vi "combine clusters (SubVI).vi"(10 "Output Configuration":T1[](array[typedef]) {"boolean high" format="%#_17g"; "boolean low" format="%#_17g"; "scan step" format="%#_17g"; "scan begin" format="%#_17g"; "scan end" format="%#_17g"}, 11 "Array in":bool[](array[boolean])) -> (3 "Array out":T2(array[cluster]))   [LabVIEW 2016]
uses:
  output configuration.ctl
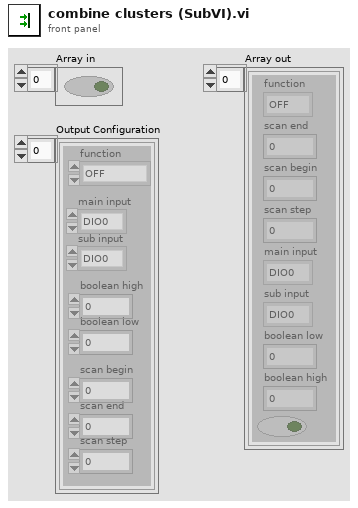
[diagram p1: front panel]
types:
  T1 = typedef "output configuration.ctl" = cluster{"function":enum16{"OFF", "SWITCH", "AND GATE", "OR GATE", "ITERATION"}, "scan end":sgl, "scan begin":sgl, "scan step":sgl, "main input":enum16{"DIO0", "DIO1", "DIO2", "DIO3", "DIO4", "DIO5", "DIO6", "DIO7", "DIO8", "DIO9", "DIO10", "DIO11", "DIO12", "DIO13", "DIO14", "DIO15", "DIO16", "DIO17", "DIO18", "DIO19", "DIO20", "DIO21", "DIO22", "DIO23", "DIO24", "DIO25", "DIO26", "DIO27", "DIO28", "DIO29", "DIO30", "DIO31"}, "sub input":enum16{"DIO0", "DIO1", "DIO2", "DIO3", "DIO4", "DIO5", "DIO6", "DIO7", "DIO8", "DIO9", "DIO10", "DIO11", "DIO12", "DIO13", "DIO14", "DIO15", "DIO16", "DIO17", "DIO18", "DIO19", "DIO20", "DIO21", "DIO22", "DIO23", "DIO24", "DIO25", "DIO26", "DIO27", "DIO28", "DIO29", "DIO30", "DIO31"}, "boolean low":sgl, "boolean high":sgl}
  T2 = cluster{"function":enum16{"OFF", "SWITCH", "AND GATE", "OR GATE", "ITERATION"}, "scan end":sgl, "scan begin":sgl, "scan step":sgl, "main input":enum16{"DIO0", "DIO1", "DIO2", "DIO3", "DIO4", "DIO5", "DIO6", "DIO7", "DIO8", "DIO9", "DIO10", "DIO11", "DIO12", "DIO13", "DIO14", "DIO15", "DIO16", "DIO17", "DIO18", "DIO19", "DIO20", "DIO21", "DIO22", "DIO23", "DIO24", "DIO25", "DIO26", "DIO27", "DIO28", "DIO29", "DIO30", "DIO31"}, "sub input":enum16{"DIO0", "DIO1", "DIO2", "DIO3", "DIO4", "DIO5", "DIO6", "DIO7", "DIO8", "DIO9", "DIO10", "DIO11", "DIO12", "DIO13", "DIO14", "DIO15", "DIO16", "DIO17", "DIO18", "DIO19", "DIO20", "DIO21", "DIO22", "DIO23", "DIO24", "DIO25", "DIO26", "DIO27", "DIO28", "DIO29", "DIO30", "DIO31"}, "boolean low":sgl, "boolean high":sgl, bool}[]
  T3 = enum16{"OFF", "SWITCH", "AND GATE", "OR GATE", "ITERATION"}
  T4 = enum16{"DIO0", "DIO1", "DIO2", "DIO3", "DIO4", "DIO5", "DIO6", "DIO7", "DIO8", "DIO9", "DIO10", "DIO11", "DIO12", "DIO13", "DIO14", "DIO15", "DIO16", "DIO17", "DIO18", "DIO19", "DIO20", "DIO21", "DIO22", "DIO23", "DIO24", "DIO25", "DIO26", "DIO27", "DIO28", "DIO29", "DIO30", "DIO31"}
  T5 = cluster{"function":enum16{"OFF", "SWITCH", "AND GATE", "OR GATE", "ITERATION"}, sgl, "scan begin":sgl, "scan step":sgl, "main input":enum16{"DIO0", "DIO1", "DIO2", "DIO3", "DIO4", "DIO5", "DIO6", "DIO7", "DIO8", "DIO9", "DIO10", "DIO11", "DIO12", "DIO13", "DIO14", "DIO15", "DIO16", "DIO17", "DIO18", "DIO19", "DIO20", "DIO21", "DIO22", "DIO23", "DIO24", "DIO25", "DIO26", "DIO27", "DIO28", "DIO29", "DIO30", "DIO31"}, "sub input":enum16{"DIO0", "DIO1", "DIO2", "DIO3", "DIO4", "DIO5", "DIO6", "DIO7", "DIO8", "DIO9", "DIO10", "DIO11", "DIO12", "DIO13", "DIO14", "DIO15", "DIO16", "DIO17", "DIO18", "DIO19", "DIO20", "DIO21", "DIO22", "DIO23", "DIO24", "DIO25", "DIO26", "DIO27", "DIO28", "DIO29", "DIO30", "DIO31"}, "boolean low":sgl, "boolean high":sgl, bool}
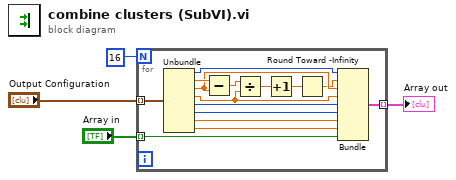
[diagram p0: block diagram]
diagram:
  n1 = for {
    N: 16 -> [_]
    tunnel: "Output Configuration" -> [w19] mode=indexing
    tunnel: "Array in" -> [w12] mode=indexing
    tunnel: [w13] -> w4 mode=indexing
    n2 = Unbundle(w19) -> ("function"=w18:T3, "scan end"=w11:sgl, "scan begin"=w10:sgl, "scan step"=w8:sgl, "main input"=w17:T4, "sub input"=w16:T4, "boolean low"=w15:sgl, "boolean high"=w14:sgl)
    n3 = Subtract(x=w11, y=w10) -> (x-y=w9:sgl)
    n4 = Divide(x=w9, y=w8) -> (x/y=w7:sgl)
    n5 = Increment(x=w7) -> (x+1=w6:sgl)
    n6 = Round Toward -Infinity(1:w6) -> (0:w5:sgl)
    n7 = Bundle("function"=w18, w5, "scan begin"=w10, "scan step"=w8, "main input"=w17, "sub input"=w16, "boolean low"=w15, "boolean high"=w14, w12) -> (w13:T5)  [unwired: 1 in]
  }
  "Array out" <- w4
